vi "MultiFileDocument.vi"(5 "Number of points":dbl, 7 "Number of sensors":dbl, 9 "Aquire Data":bool, 10 "Multivalues":sgl[][][](array[numeric]), 11 "File Path In":path) -> (3 "file path out":path)   [LabVIEW 2019]
uses:
  <vilib>/Utility/file.llb/Write Delimited Spreadsheet (string).vi
  <vilib>/Utility/file.llb/Write Delimited Spreadsheet (DBL).vi
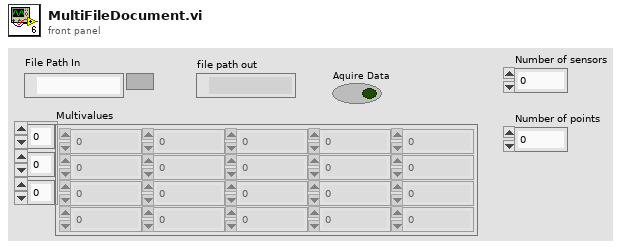
[diagram p1: front panel]
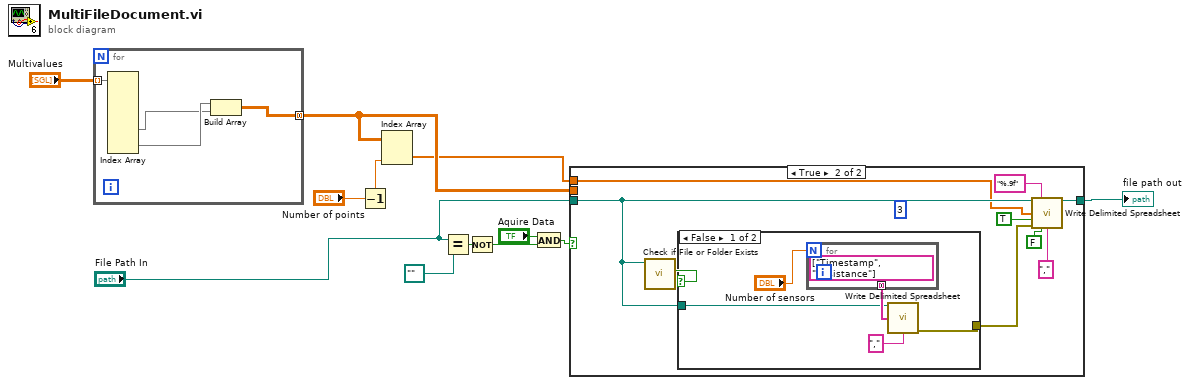
[diagram p0: block diagram]
diagram:
  n1 = for {
    tunnel: [w14] -> w4 mode=concatenating
    tunnel: "Multivalues" -> [w16] mode=indexing
    n2 = Index Array(array=w16) -> (element #3=w13:sgl[], element #4=w15:sgl[])  [unwired: 8 in, 2 out]
    n3 = Build Array(w15, w13) -> (w14:sgl[][])
  }
  n4 = Decrement(x="Number of points") -> (x-1=w1:dbl)
  n5 = Index Array(array=w4, index (col)=w1) -> (element=w3:sgl[])  [unwired: 1 in]
  n6 = Equal?(x="File Path In", y=path "") -> (x = y?=w6:bool)
  n7 = Not(x=w6) -> (.not. x?=w10:bool)
  n8 = And(x="Aquire Data", y=w10) -> (x .and. y?=w12:bool)
  n9 = case shown="True" w12 {
    tunnel: [w17 w26] -> w9
    tunnel: "File Path In" -> [w17 w22]
    tunnel: w4 -> [_ _]
    tunnel: w3 -> [_ w18]
    frame False {
    }
    frame True {
      (unwired) 3 ("index (row)")
      n10 = call <vilib>:"Check if File or Folder Exists.vi"("path"=w22) -> ("file or folder exists?"=w23:bool)  [unwired: 8 in, 2 out]
      n11 = case shown="False" w23 {
        tunnel: w22 -> [w30 _]
        tunnel: [w29 _] -> w21
        frame False {
          n12 = for {
            N: "Number of sensors" -> [_]
            tunnel: [string[] ["Timestamp", "Resistance"] ("1D data")] -> w31 mode=concatenating
          }
          n13 = call-poly <vilib>:"Write Delimited Spreadsheet.vi"("file path (dialog if empty)"=w30, "1D data"=w31, "delimiter (\\t)"="," ("delimiter (\\t)")) -> ("error out"=w29:errorcluster)  [unwired: 11 in, 1 out]
        }
        frame True {
        }
      }
      n14 = call-poly <vilib>:"Write Delimited Spreadsheet.vi"("file path (dialog if empty)"=w22, "format (%.3f)"="%.9f" ("format (%s)"), "1D data"=w18, "append to file? (new file:F)"=TRUE, "error in (no error)"=w21, "transpose? (no:F)"=FALSE, "delimiter (\\t)"="," ("delimiter (\\t)")) -> ("new file path (Not A Path if cancelled)"=w26:path)  [unwired: 7 in, 1 out]
    }
  }
  "file path out" <- w9
